vi "SVT Vibration Level.vi"   [LabVIEW 2017, in "SoundVib_VibrationLevel.lvlib"]
doc: "Computes several vibration level measurements including the root-mean-square (RMS) level, running RMS level, exponential averaged level, peak level, and max-min level. Each instance of this VI maintains its own state; use the N Channel instance of this VI to process an array of channels. This VI operates on time-continuous data; it resets on a discontinuity.<B> Scaled signal [EU]</B> should have a zero DC component. You can attenuate the DC component with hardware AC-coupling filters and with software high-pass filters. Wire data to the <B> scaled signal [EU]</B> input to determine the polymorphic instance to use or manually select the instance."
uses:
  <vilib>/addons/Sound and Vibration/svt_Level/SoundVib_VibrationLevel.lvlib
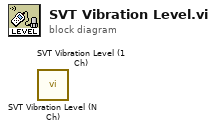
[diagram p0: block diagram]
diagram:
  n1 = call <vilib>:"SVT Vibration Level (N Ch).vi"() -> ()  [unwired: 9 in, 7 out]
  n2 = call <vilib>:"SVT Vibration Level (1 Ch).vi"() -> ()  [unwired: 9 in, 7 out]
